vi "Defer_FP_Updates.vi"(7 "Defer Panel Updates":bool, 8 "error in":errorcluster, 11 "lv_icon.vi in":refnum<vi>) -> (0 "error out":errorcluster, 3 "lv icon.vi out":refnum<vi>)   [LabVIEW 2021]
doc: "Applys or removes the Defer Panel Updates to the panel of lv_icon.vi."
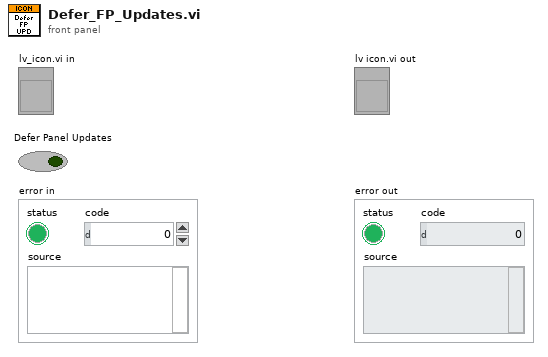
[diagram p1: front panel]
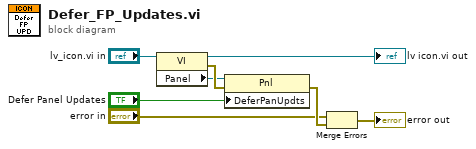
[diagram p0: block diagram]
diagram:
  n1 = property class="VI"(reference="lv_icon.vi in") -> (reference out=→"lv icon.vi out":refnum<vi>, error out=w6:errorcluster, "Panel"=w4:refnum<vi>)  [unwired: 1 in]
  n2 = property class="Pnl"(reference=w4, error in=w6, "DeferPanUpdts"="Defer Panel Updates") -> (error out=w8:errorcluster)  [unwired: 1 out]
  n3 = Merge Errors("error in", w8) -> (→"error out":errorcluster)
